vi "DriveStraightforDistance-2.vi"(6 "Y axis speed":dbl, 7 "Target Angle":dbl, 9 "X axis speed":dbl, 10 "Distance to travel":dbl, 11 "RobotDriveDevRef":T1) -> ()   [LabVIEW 2017]
uses:
  <vilib>/Rock Robotics/WPI/RobotDrive/WPI_RobotDriveDevRef.ctl
  <vilib>/Rock Robotics/WPI/MotorControl/WPI_MotorControlDeviceRef.ctl
  <vilib>/Rock Robotics/WPI/MotorControl/WPI_MotorControlType.ctl
  <vilib>/Rock Robotics/SystemInterfaces/DIO/FPGA_DIOPWMChannel.ctl
  <vilib>/Rock Robotics/WPI/PWM/WPI_PWMDeadband.ctl
  <vilib>/Rock Robotics/SystemInterfaces/DIO/FPGA_DIOChannel.ctl
  Robot Global Data.vi
  <vilib>/addons/control/pid/pid.llb/PID (DBL).vi
  <vilib>/Rock Robotics/WPI/RobotDrive/WPI_RobotDriveArcadeDrive_Standard(NoSaturation).vi
  <vilib>/addons/control/pid/NI_PID_pid.lvlib
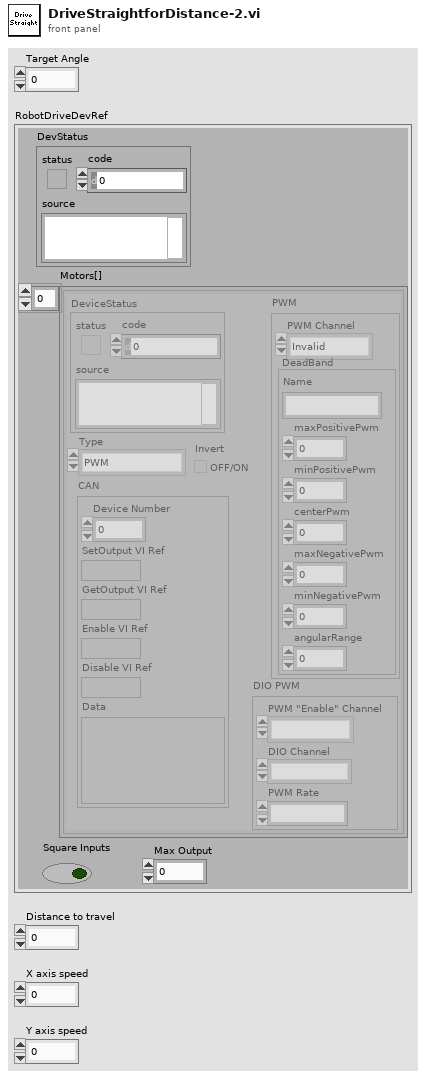
[diagram p1: front panel]
types:
  T1 = typedef "WPI_RobotDriveDevRef.ctl" = cluster{"DevStatus":errorcluster, "Motors[]":T2[], "Square Inputs":bool, "Max Output":dbl}
  T2 = typedef "WPI_MotorControlDeviceRef.ctl" = cluster{"DeviceStatus":errorcluster, "Type":T3, "PWM":cluster{"PWM Channel":T4, "DeadBand":T5}, "CAN":cluster{"Device Number":u8, "SetOutput VI Ref":variant, "GetOutput VI Ref":variant, "Enable VI Ref":variant, "Disable VI Ref":variant, "Data":variant}, "Invert":bool, "DIO PWM":cluster{"PWM \"Enable\" Channel":T4, "DIOChannel":T6, "PWM Rate":dbl}}
  T3 = typedef "WPI_MotorControlType.ctl" = enum16{"PWM", "CAN", "DIO PWM"}
  T4 = typedef "FPGA_DIOPWMChannel.ctl" = enum8{"PWM 0", "PWM 1", "PWM 2", "PWM 3", "PWM 4", "PWM 5", "PWM 6", "PWM 7", "PWM 8", "PWM 9", "PWM MXP 0", "PWM MXP 1", "PWM MXP 2", "PWM MXP 3", "PWM MXP 4", "PWM MXP 5", "PWM MXP 6", "PWM MXP 7", "PWM MXP 8", "PWM MXP 9", "Invalid"}
  T5 = typedef "WPI_PWMDeadband.ctl" = cluster{"Name":string, "maxPositivePwm":i32, "minPositivePwm":i32, "centerPwm":i32, "maxNegativePwm":i32, "minNegativePwm":i32, "angularRange":u16}
  T6 = typedef "FPGA_DIOChannel.ctl" = enum8{"DIO 0", "DIO 1", "DIO 2", "DIO 3", "DIO 4", "DIO 5", "DIO 6", "DIO 7", "DIO 8", "DIO 9", "DIO MXP 0", "DIO MXP 1", "DIO MXP 2", "DIO MXP 3", "DIO MXP 4", "DIO MXP 5", "DIO MXP 6", "DIO MXP 7", "DIO MXP 8", "DIO MXP 9", "DIO MXP 10", "DIO MXP 11", "DIO MXP 12", "DIO MXP 13", "DIO MXP 14", "DIO MXP 15", "SPI Port CS1", "SPI Port CS2", "SPI Port CS3", "SPI Port MISO", "SPI Port MOSI", "Invalid"}
  T7 = cluster{"proportional gain (Kc)":dbl, "integral time (Ti, min)":dbl, "derivative time (Td, min)":dbl}
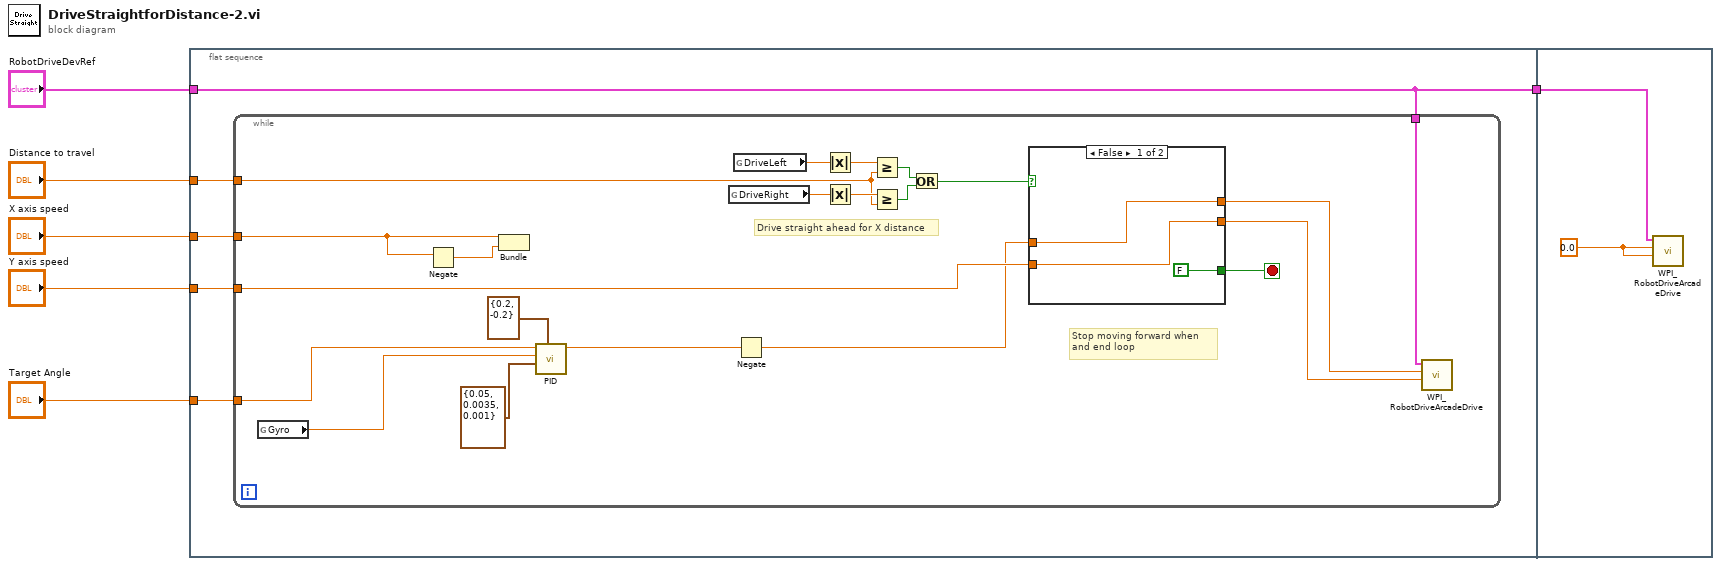
[diagram p0: block diagram]
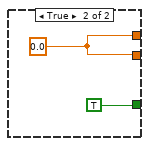
[diagram p2: hidden frame]
diagram:
  n1 = flat-sequence {
    tunnel: "RobotDriveDevRef" -> [w11]
    tunnel: [w11] -> w6
    tunnel: "Distance to travel" -> [w10]
    tunnel: "X axis speed" -> [w9]
    tunnel: "Y axis speed" -> [w8]
    tunnel: "Target Angle" -> [w7]
    tunnel: w6 -> [w38]
    frame #0 {
      n2 = while {
        tunnel: w11 -> [w22]
        tunnel: w10 -> [w21]
        tunnel: w9 -> [w14]
        tunnel: w8 -> [w20]
        tunnel: w7 -> [w18]
        stop <- w26 stop-if-true
        # "Stop moving forward when\nand end loop"
        # "Drive straight ahead for X distance"
        n3 = global read "Robot Global Data.vi" "Gyro"() -> (w17:dbl)
        n4 = Negate(x=w14) -> (-x=w15:dbl)
        n5 = Bundle("X axis speed"=w14, w15) -> ()  [unwired: 1 in, 1 out]
        n6 = call-poly <vilib>:"PID.vi"("output range"=cluster{"output high":dbl, "output low":dbl} {"output high"=0.2, "output low"=-0.2}, "PID gains"=T7 {"proportional gain (Kc)"=0.05, "integral time (Ti, min)"=0.0035, "derivative time (Td, min)"=0.001}, "process variable"=w17, "setpoint"=w18) -> ("output"=w19:dbl)  [unwired: 6 in, 1 out]
        n7 = global read "Robot Global Data.vi" "DriveRight"() -> (w24:dbl)
        n8 = global read "Robot Global Data.vi" "DriveLeft"() -> (w23:dbl)
        n9 = Negate(x=w19) -> (-x=w12:dbl)
        n10 = Absolute Value(x=w23) -> (abs(x)=w29:dbl)
        n11 = Absolute Value(x=w24) -> (abs(x)=w30:dbl)
        n12 = Greater Or Equal?(x=w29, y=w21) -> (x >= y?=w32:bool)
        n13 = Greater Or Equal?(x=w30, y=w21) -> (x >= y?=w31:bool)
        n14 = Or(x=w32, y=w31) -> (x .or. y?=w25:bool)
        n15 = case shown="False" w25 {
          tunnel: [w35 w37] -> w27
          tunnel: [w33 w37] -> w28
          tunnel: w20 -> [w33 _]
          tunnel: w12 -> [w35 _]
          tunnel: [FALSE TRUE] -> w26
          frame False {
          }
          frame True {
            w37 = 0.0
          }
        }
        n16 = call-poly <vilib>:"WPI_RobotDriveArcadeDrive.vi"("Y axis value"=w28, "X axis value"=w27, "RobotDriveDevRef"=w22) -> ()  [unwired: 6 in, 3 out]
      }
    }
    frame #1 {
      w39 = 0.0 ("X axis value")
      n17 = call-poly <vilib>:"WPI_RobotDriveArcadeDrive.vi"("Y axis value"=w39, "X axis value"=w39, "RobotDriveDevRef"=w38) -> ()  [unwired: 6 in, 3 out]
    }
  }
